vi "Security.vi"(8 "Error In":errorcluster, 11 "User Creds":T1) -> (0 "error out":errorcluster)   [LabVIEW 2023]
uses:
  UsersList.ctl
  UserCredentials.ctl
  QSM - Security/Controls/State Machine Message.ctl
  QSM - Security/Controls/Message Queue Element Position.ctl
  QSM - Security/QSM - Security.lvlib
panel:
  in  "Save User":bool
  in  "Edit User":bool
  in  "Remove User":bool
  in  "Close":bool
  in  "Save Button":bool
  in  "User Permissions":T2
  # "USER PERMISSIONS"
  # "** To Edit User Permissions:\n- Select the row of the user\nyou wish to edit.\n- Press the \"Edit User\" button\n- Make desired changes\n- Press \"SAVE\" button,\notherwise changes will not\nbe saved."
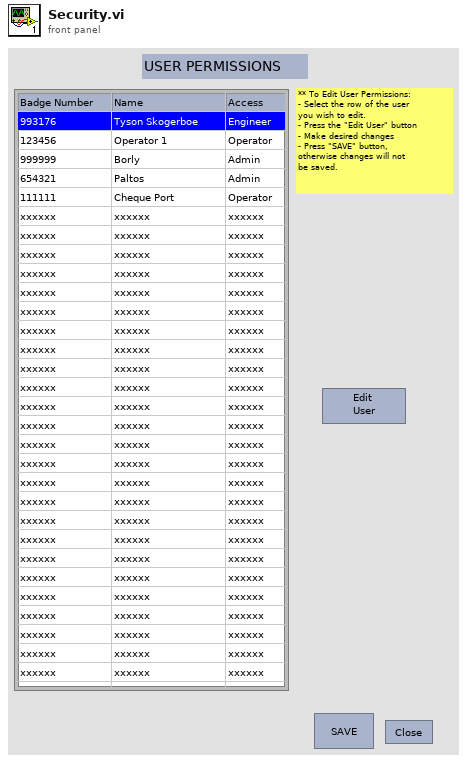
[diagram p1: front panel]
types:
  T1 = typedef "UserCredentials.ctl" = cluster{"Badge Number":string, "Name":string, "Access":enum16{"", "Operator", "Admin", "Engineer"}}
  T2 = typedef "UsersList.ctl" = i32
  T3 = typedef "QSM - Security.lvlib/State Machine Message.ctl" = enum16{"Initialize", "Save Button", "Save User", "Remove User", "Edit User", "Handle Error", "Exit"}
  T4 = typedef "QSM - Security.lvlib/Message Queue Element Position.ctl" = enum16{"Front", "Back"}
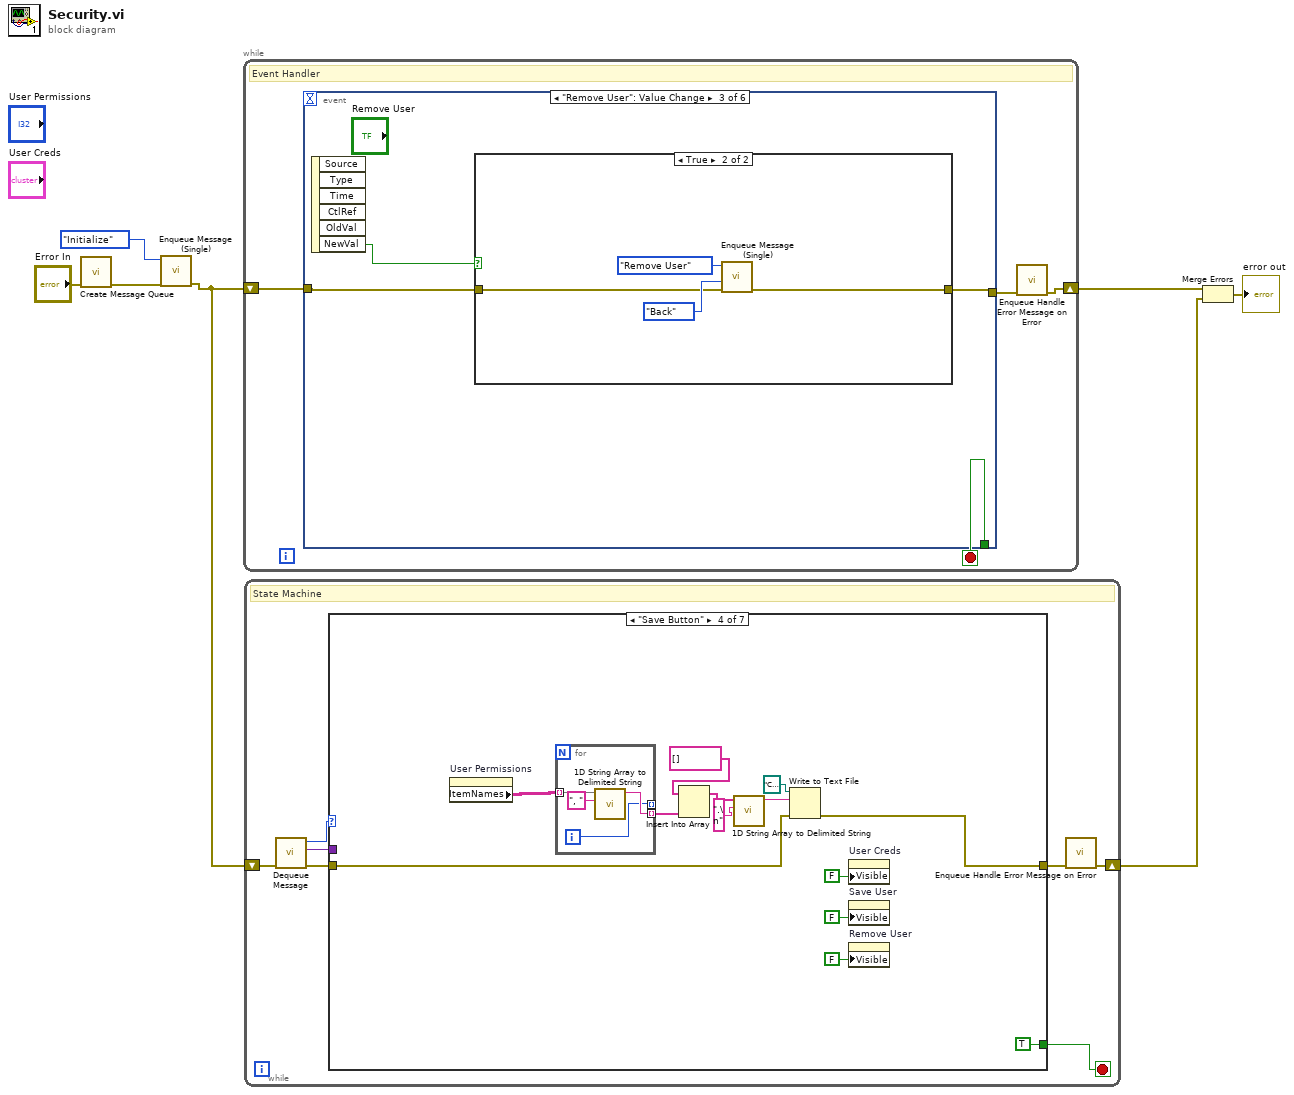
[diagram p0: block diagram]
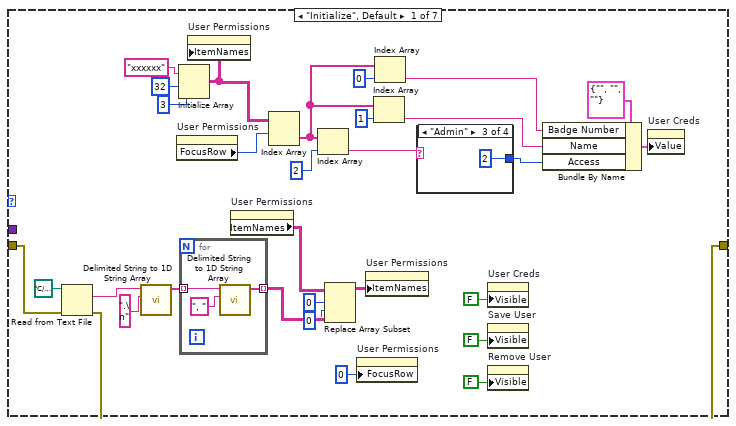
[diagram p2: hidden frame]
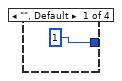
[diagram p3: hidden frame]
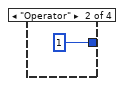
[diagram p4: hidden frame]
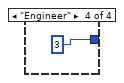
[diagram p5: hidden frame]
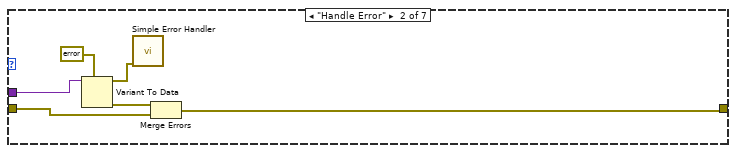
[diagram p6: hidden frame]
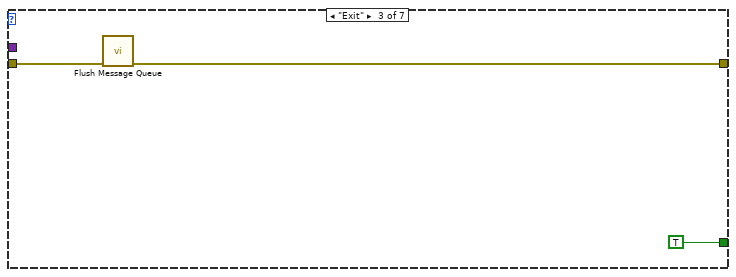
[diagram p7: hidden frame]
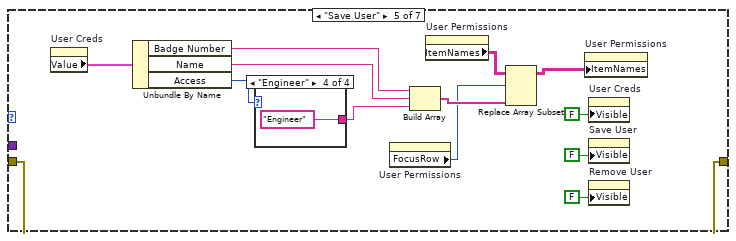
[diagram p8: hidden frame]
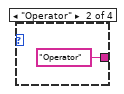
[diagram p10: hidden frame]
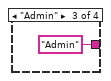
[diagram p11: hidden frame]
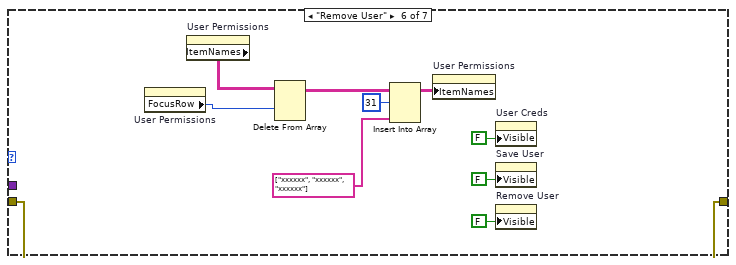
[diagram p12: hidden frame]
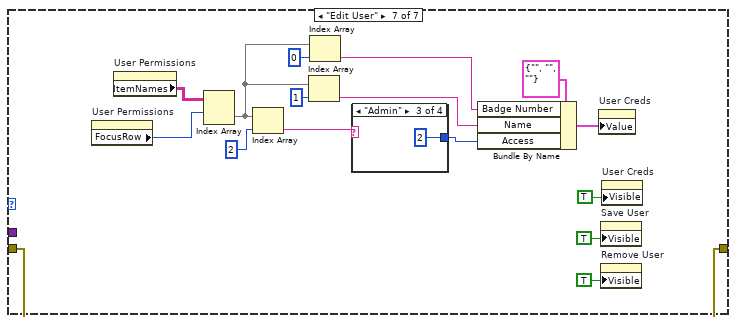
[diagram p13: hidden frame]
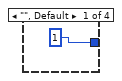
[diagram p14: hidden frame]
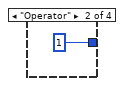
[diagram p15: hidden frame]
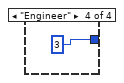
[diagram p16: hidden frame]
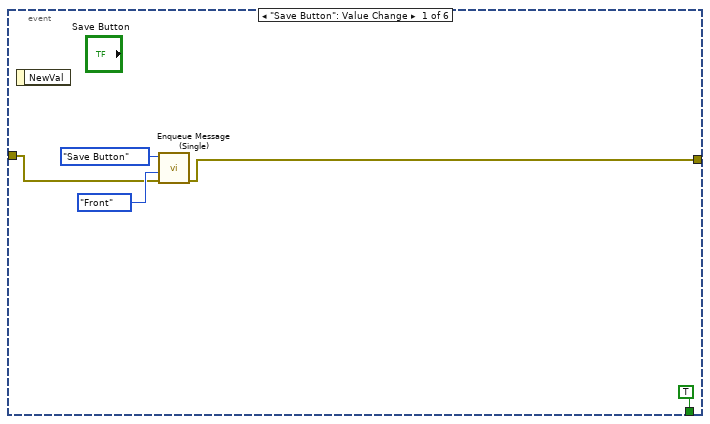
[diagram p17: hidden frame]
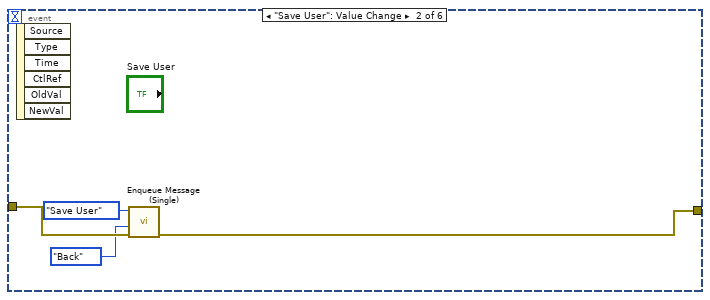
[diagram p18: hidden frame]
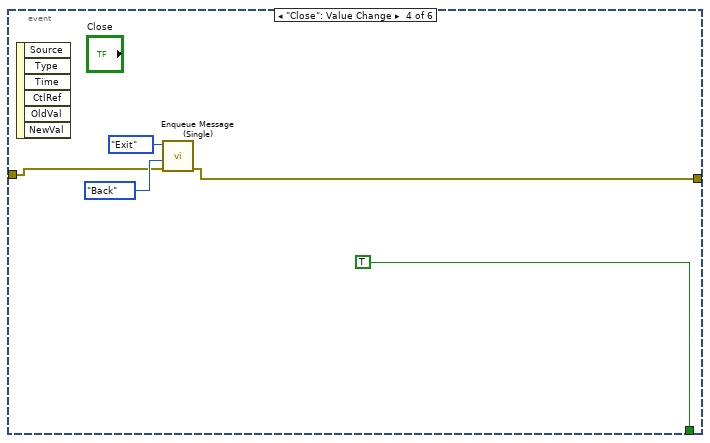
[diagram p20: hidden frame]
diagram:
  n1 = call "Create Message Queue.vi"("Error In"="Error In") -> ("Error Out"=w7:errorcluster)  [unwired: 10 in]
  n2 = call "Enqueue Message (Single).vi"("Error In"=w7, "State Machine Message"=State_Machine_Message."Initialize") -> ("Error Out"=w5:errorcluster)  [unwired: 9 in]
  n3 = while {
    shift-right: [w10] -> w4
    shift-left: w5 -> [w8]
    stop <- w11 stop-if-true
    # "Event Handler"
    n4 = event shown="[2] \"Remove User\": Value Change" {
      selector: _ -> [_ _ _ _ _ _]
      dyn-events: _ -> [_ _ _ _ _ _]
      timeout: _ -> [_ _ _ _ _ _]
      tunnel: [TRUE _ _ TRUE _ _] -> w11
      tunnel: [w13 w17 w21 w29 w34 w39] -> w9
      tunnel: w8 -> [w14 w20 w22 w30 w35 w40]
      event "Save Button": Value Change {
        n5 = event-data() -> ()  [unwired: 1 in, 1 out]
        n6 = call "Enqueue Message (Single).vi"("Error In"=w14, "Message Position"=Message_Queue_Element_Position."Front", "State Machine Message"=State_Machine_Message."Save Button") -> ("Error Out"=w13:errorcluster)  [unwired: 8 in]
      }
      event "Save User": Value Change {
        n7 = event-data() -> ()  [unwired: 1 in, 6 out]
        n8 = call "Enqueue Message (Single).vi"("Error In"=w20, "Message Position"=Message_Queue_Element_Position."Back", "State Machine Message"=State_Machine_Message."Save User") -> ("Error Out"=w17:errorcluster)  [unwired: 8 in]
      }
      event "Remove User": Value Change {
        n9 = event-data() -> ("NewVal"=w23:bool)  [unwired: 1 in, 5 out]
        n10 = case shown="True" w23 {
          tunnel: w22 -> [w24 w26]
          tunnel: [w24 w25] -> w21
          frame False {
          }
          frame True {
            n11 = call "Enqueue Message (Single).vi"("Error In"=w26, "Message Position"=Message_Queue_Element_Position."Back", "State Machine Message"=State_Machine_Message."Remove User") -> ("Error Out"=w25:errorcluster)  [unwired: 8 in]
          }
        }
      }
      event "Close": Value Change {
        n12 = event-data() -> ()  [unwired: 1 in, 6 out]
        n13 = call "Enqueue Message (Single).vi"("Error In"=w30, "Message Position"=Message_Queue_Element_Position."Back", "State Machine Message"=State_Machine_Message."Exit") -> ("Error Out"=w29:errorcluster)  [unwired: 8 in]
      }
      event "Edit User": Value Change {
        n14 = event-data() -> ()  [unwired: 1 in, 6 out]
        n15 = call "Enqueue Message (Single).vi"("Error In"=w35, "Message Position"=Message_Queue_Element_Position."Back", "State Machine Message"=State_Machine_Message."Edit User") -> ("Error Out"=w34:errorcluster)  [unwired: 8 in]
      }
      event Double Click {
        n16 = event-data() -> ("Row"=w38:i32)  [unwired: 1 in, 8 out]
        n17 = property on="User Permissions" class="MCListbox (strict)"("FocusRow"=w38) -> ()  [unwired: 2 in, 2 out]
        n18 = call "Enqueue Message (Single).vi"("Error In"=w40, "Message Position"=Message_Queue_Element_Position."Back", "State Machine Message"=State_Machine_Message."Edit User") -> ("Error Out"=w39:errorcluster)  [unwired: 8 in]
      }
    }
    n19 = call "Enqueue Handle Error Message on Error.vi"("Error In"=w9) -> ("Error Out"=w10:errorcluster)  [unwired: 10 in]
  }
  n20 = while {
    shift-right: [w48] -> w3
    shift-left: w5 -> [w49]
    stop <- w43 stop-if-true
    # "State Machine"
    n21 = call "Dequeue Message.vi"("Error In"=w49) -> ("Error Out"=w47:errorcluster, "Data"=w46:variant, "State Machine Message"=w45:T3)  [unwired: 8 in]
    n22 = case shown="\"Save Button\"" w45 {
      tunnel: w47 -> [w52 w88 w95 w98 w115 w129 w139]
      tunnel: w46 -> [_ w92 _ _ _ _ _]
      tunnel: [w51 w87 w94 w97 w115 w129 w139] -> w44
      tunnel: [_ _ TRUE TRUE _ _ _] -> w43
      frame "Initialize", Default {
        n23 = Read from Text File(file (use dialog)=path "C:/Users/Public/Documents/Grid2093/Security/Permissions.txt", error in=w52) -> (text=w64:string, error out=w51:errorcluster)  [unwired: 2 in, 2 out]
        n24 = call <vilib>:"Delimited String to 1D String Array.vi"("delimiter"=".\n", "delimited string"=w64) -> ("string array"=w65:string[])  [unwired: 9 in]
        n25 = property on="User Permissions" class="MCListbox (strict)"() -> ("FocusRow"=w66:i32)  [unwired: 2 in, 2 out]
        n26 = Initialize Array("xxxxxx", 32 ("dimension size"), 3 ("dimension size")) -> (w73:string[][])
        n27 = for {
          tunnel: w65 -> [w86] mode=indexing
          tunnel: [w84] -> w76 mode=indexing
          n28 = call <vilib>:"Delimited String to 1D String Array.vi"("delimiter"=", ", "delimited string"=w86) -> ("string array"=w84:string[])  [unwired: 9 in]
        }
        n29 = property on="User Permissions" class="MCListbox (strict)"("ItemNames"=w73) -> ()  [unwired: 2 in, 2 out]
        n30 = property on="User Permissions" class="MCListbox (strict)"() -> ("ItemNames"=w74:string[][])  [unwired: 2 in, 2 out]
        n31 = Index Array(array=w73, index (row)=w66) -> (element=w70:string[])  [unwired: 1 in]
        n32 = Index Array(array=w70, index=2) -> (element=w67:string)
        n33 = Replace Array Subset(array=w74, new element=w76, index (row)=0, index (col)=0 ("disabled index (col)")) -> (w75:string[][])
        n34 = property on="User Permissions" class="MCListbox (strict)"("FocusRow"=0 ("Focus Row")) -> ()  [unwired: 2 in, 2 out]
        n35 = property on="User Permissions" class="MCListbox (strict)"("ItemNames"=w75) -> ()  [unwired: 2 in, 2 out]
        n36 = Index Array(array=w70, index=1) -> (element=w69:string)
        n37 = Index Array(array=w70, index=0) -> (element=w71:string)
        n38 = case shown="\"Admin\"" w67 {
          tunnel: [u16 1 ("Access") u16 1 ("Access") u16 2 ("Access") u16 3 ("Access")] -> w68
          frame "", Default {
          }
          frame "Operator" {
          }
          frame "Admin" {
          }
          frame "Engineer" {
          }
        }
        n39 = property on="User Creds" class="Clust (strict)"("Visible"=FALSE) -> ()  [unwired: 2 in, 2 out]
        n40 = property on="Save User" class="Bool (strict)"("Visible"=FALSE) -> ()  [unwired: 2 in, 2 out]
        n41 = property on="Remove User" class="Bool (strict)"("Visible"=FALSE) -> ()  [unwired: 2 in, 2 out]
        n42 = Bundle By Name(cluster=T1 {"Badge Number"="", "Name"="", "Access"=enum.""} ("User Creds"), "Badge Number"=w71, "Name"=w69, "Access"=w68) -> (w72:T1)
        n43 = property on="User Creds" class="Clust (strict)"("Value"=w72) -> ()  [unwired: 2 in, 2 out]
      }
      frame "Handle Error" {
        n44 = Variant To Data(type=errorcluster {"status"=FALSE, "code"=0, "source"=""} ("Error In"), Variant=w92) -> (data=w90:errorcluster, error out=w89:errorcluster)  [unwired: 1 in]
        n45 = call <vilib>:"Simple Error Handler.vi"("error in (no error)"=w90) -> ()  [unwired: 4 in, 5 out]
        n46 = Merge Errors(w89, w88) -> (w87:errorcluster)
      }
      frame "Exit" {
        n47 = call "Flush Message Queue.vi"("Error In"=w95) -> ("Error Out"=w94:errorcluster)  [unwired: 9 in, 1 out]
      }
      frame "Save Button" {
        n48 = property on="User Permissions" class="MCListbox (strict)"() -> ("ItemNames"=w108:string[][])  [unwired: 2 in, 2 out]
        n49 = for {
          tunnel: w108 -> [w112] mode=indexing
          tunnel: [w110] -> w105 mode=indexing
          tunnel: [w109] -> _ mode=indexing
          i -> [w109]
          n50 = call <vilib>:"1D String Array to Delimited String.vi"("delimiter"=", ", "string array"=w112) -> ("delimited string"=w110:string)  [unwired: 9 in]
        }
        n51 = Insert Into Array(array=string[] [] ("string array"), new element=w105) -> (w106:string[])  [unwired: 1 in]
        n52 = call <vilib>:"1D String Array to Delimited String.vi"("delimiter"=".\n", "string array"=w106) -> ("delimited string"=w107:string)  [unwired: 9 in]
        n53 = Write to Text File(file (use dialog)=path "C:/Users/Public/Documents/Grid2093/Security/Permissions.txt", text=w107, error in=w98) -> (error out=w97:errorcluster)  [unwired: 1 in, 2 out]
        n54 = property on="User Creds" class="Clust (strict)"("Visible"=FALSE) -> ()  [unwired: 2 in, 2 out]
        n55 = property on="Save User" class="Bool (strict)"("Visible"=FALSE) -> ()  [unwired: 2 in, 2 out]
        n56 = property on="Remove User" class="Bool (strict)"("Visible"=FALSE) -> ()  [unwired: 2 in, 2 out]
      }
      frame "Save User" {
        n57 = property on="User Creds" class="Clust (strict)"() -> ("Value"=w113:T1)  [unwired: 2 in, 2 out]
        n58 = Unbundle By Name(w113) -> ("Badge Number"=w124:string, "Name"=w123:string, "Access"=w114:enum16{"", "Operator", "Admin", "Engineer"})
        n59 = case shown="\"Engineer\"" w114 {
          tunnel: [_ "Operator" "Admin" "Engineer"] -> w122
          frame "", Default {
          }
          frame "Operator" {
          }
          frame "Admin" {
          }
          frame "Engineer" {
          }
        }
        n60 = property on="User Permissions" class="MCListbox (strict)"() -> ("FocusRow"=w119:i32)  [unwired: 2 in, 2 out]
        n61 = Build Array(w124, w123, w122) -> (w120:string[])
        n62 = property on="User Permissions" class="MCListbox (strict)"() -> ("ItemNames"=w121:string[][])  [unwired: 2 in, 2 out]
        n63 = Replace Array Subset(array=w121, new element=w120, index (row)=w119) -> (w125:string[][])  [unwired: 1 in]
        n64 = property on="User Permissions" class="MCListbox (strict)"("ItemNames"=w125) -> ()  [unwired: 2 in, 2 out]
        n65 = property on="User Creds" class="Clust (strict)"("Visible"=FALSE) -> ()  [unwired: 2 in, 2 out]
        n66 = property on="Save User" class="Bool (strict)"("Visible"=FALSE) -> ()  [unwired: 2 in, 2 out]
        n67 = property on="Remove User" class="Bool (strict)"("Visible"=FALSE) -> ()  [unwired: 2 in, 2 out]
      }
      frame "Remove User" {
        n68 = property on="User Permissions" class="MCListbox (strict)"() -> ("FocusRow"=w136:i32)  [unwired: 2 in, 2 out]
        n69 = property on="User Permissions" class="MCListbox (strict)"() -> ("ItemNames"=w135:string[][])  [unwired: 2 in, 2 out]
        n70 = Delete From Array(array=w135, index (row)=w136) -> (array with subset deleted=w137:string[][])  [unwired: 2 in, 1 out]
        n71 = Insert Into Array(array=w137, index (row)=31, new element=string[] ["xxxxxx", "xxxxxx", "xxxxxx"] ("new element/subarray")) -> (w138:string[][])  [unwired: 1 in]
        n72 = property on="User Permissions" class="MCListbox (strict)"("ItemNames"=w138) -> ()  [unwired: 2 in, 2 out]
        n73 = property on="User Creds" class="Clust (strict)"("Visible"=FALSE) -> ()  [unwired: 2 in, 2 out]
        n74 = property on="Save User" class="Bool (strict)"("Visible"=FALSE) -> ()  [unwired: 2 in, 2 out]
        n75 = property on="Remove User" class="Bool (strict)"("Visible"=FALSE) -> ()  [unwired: 2 in, 2 out]
      }
      frame "Edit User" {
        n76 = property on="User Permissions" class="MCListbox (strict)"() -> ("FocusRow"=w154:i32)  [unwired: 2 in, 2 out]
        n77 = property on="User Permissions" class="MCListbox (strict)"() -> ("ItemNames"=w152:string[][])  [unwired: 2 in, 2 out]
        n78 = Index Array(array=w152, index (row)=w154) -> (element=w148:string[])  [unwired: 1 in]
        n79 = Index Array(array=w148, index=2) -> (element=w151:string)
        n80 = Index Array(array=w148, index=1) -> (element=w149:string)
        n81 = Index Array(array=w148, index=0) -> (element=w147:string)
        n82 = case shown="\"Admin\"" w151 {
          tunnel: [u16 1 ("Access") u16 1 ("Access") u16 2 ("Access") u16 3 ("Access")] -> w150
          frame "", Default {
          }
          frame "Operator" {
          }
          frame "Admin" {
          }
          frame "Engineer" {
          }
        }
        n83 = Bundle By Name(cluster=T1 {"Badge Number"="", "Name"="", "Access"=enum.""} ("User Creds"), "Badge Number"=w147, "Name"=w149, "Access"=w150) -> (w153:T1)
        n84 = property on="User Creds" class="Clust (strict)"("Value"=w153) -> ()  [unwired: 2 in, 2 out]
        n85 = property on="Save User" class="Bool (strict)"("Visible"=TRUE) -> ()  [unwired: 2 in, 2 out]
        n86 = property on="Remove User" class="Bool (strict)"("Visible"=TRUE) -> ()  [unwired: 2 in, 2 out]
        n87 = property on="User Creds" class="Clust (strict)"("Visible"=TRUE) -> ()  [unwired: 2 in, 2 out]
      }
    }
    n88 = call "Enqueue Handle Error Message on Error.vi"("Error In"=w44) -> ("Error Out"=w48:errorcluster)  [unwired: 10 in]
  }
  n89 = Merge Errors(w4, w3) -> (→"error out":errorcluster)
